vi "Initialize.vi"(8 "error in (no error)":errorcluster, 11 "UDP Transfer Rx User Interface in":refnum<class "UDP Transfer Tx User Interface.lvclass">) -> (0 "error out":errorcluster, 3 "UDP Transfer Rx User Interface out":refnum<class "UDP Transfer Tx User Interface.lvclass">)   [LabVIEW 2023, in "UDP.lvlib" / "UDP Transfer Tx User Interface.lvclass"]
uses:
  UDP Transfer Tx User Interface.lvclass
  C:/Users/Public/Documents/National Instruments/NI VeriStand 2023/Custom Devices/Data Sharing Framework/Linux_x64/DSF Core.lvlibp/Classes/User Interface/User Interface.lvclass
  Configuration/Tx Transfer/UDP Transfer Tx Configuration.lvclass
  C:/Users/Public/Documents/National Instruments/NI VeriStand 2023/Custom Devices/Data Sharing Framework/Linux_x64/DSF Core.lvlibp/Classes/Configuration/Configuration.lvclass
  Users/Public/Documents/National Instruments/NI VeriStand 2023/Custom Devices/Data Sharing Framework/Linux_x64/DSF Core.lvlibp/Classes/User Interface/User Interface.lvclass
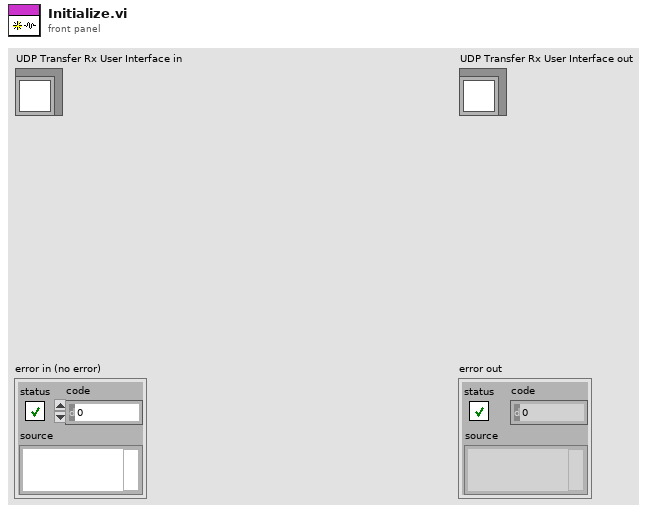
[diagram p1: front panel]
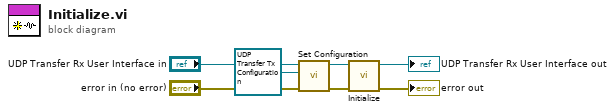
[diagram p0: block diagram]
diagram:
  n1 = call "Set Configuration.vi"("error in (no error)"="error in (no error)", "configuration"=refnum<class "UDP Transfer Tx Configuration.lvclass"> refnum ("DSF Core.lvlib:UDP Transfer Tx Configuration.lvclass"), "User Interface in"="UDP Transfer Rx User Interface in") -> ("error out"=w5:errorcluster, "User Interface out"=w4:refnum<class "UDP Transfer Tx User Interface.lvclass">)  [unwired: 7 in]
  n2 = call-parent "Initialize.vi"("error in (no error)"=w5, "User Interface in"=w4) -> ("error out"=→"error out":errorcluster, "User Interface out"=→"UDP Transfer Rx User Interface out":refnum<class "UDP Transfer Tx User Interface.lvclass">)  [unwired: 8 in]
